vi "as2_startLogFile.vi"(4 "error in (no error)":errorcluster, 6 "Path In":path) -> (0 "error out":errorcluster, 2 "Path":path)   [LabVIEW 2013]
uses:
  <vilib>/Utility/file.llb/Write To Spreadsheet File (string).vi
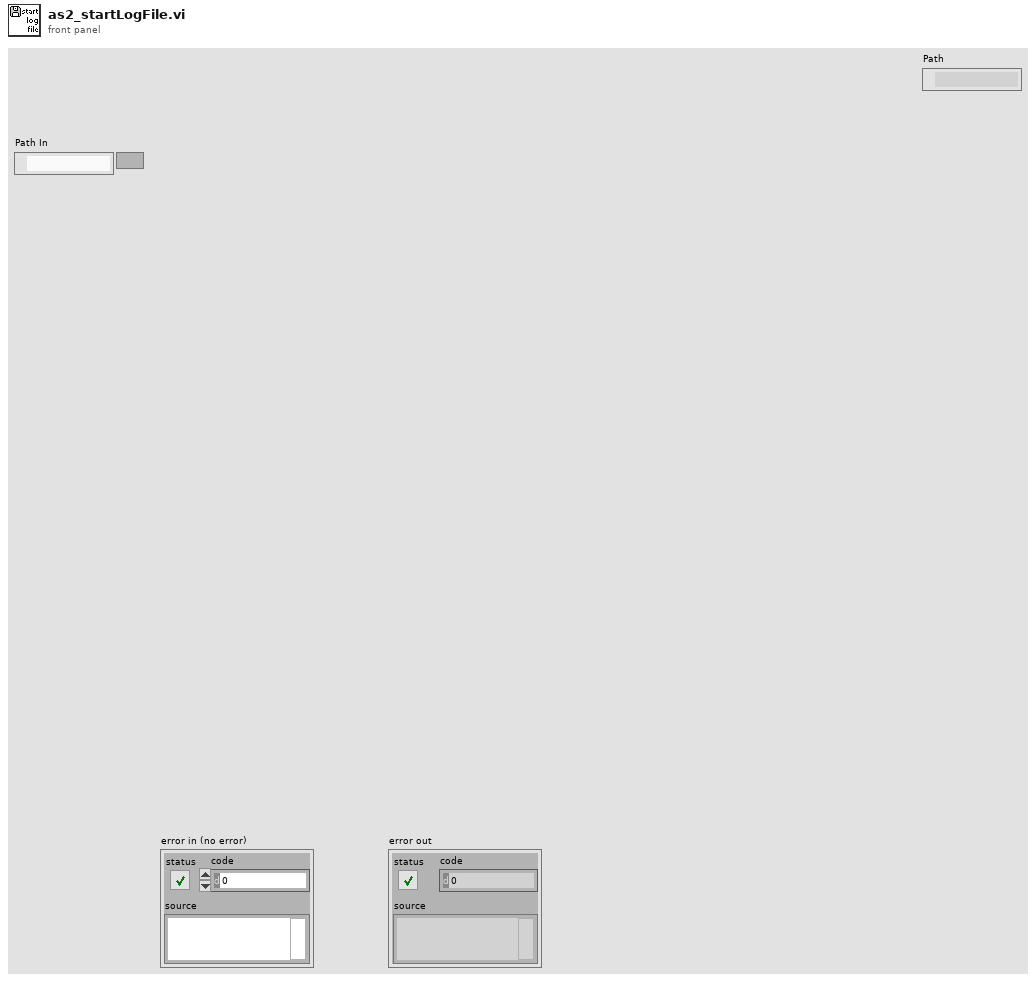
[diagram p1: front panel]
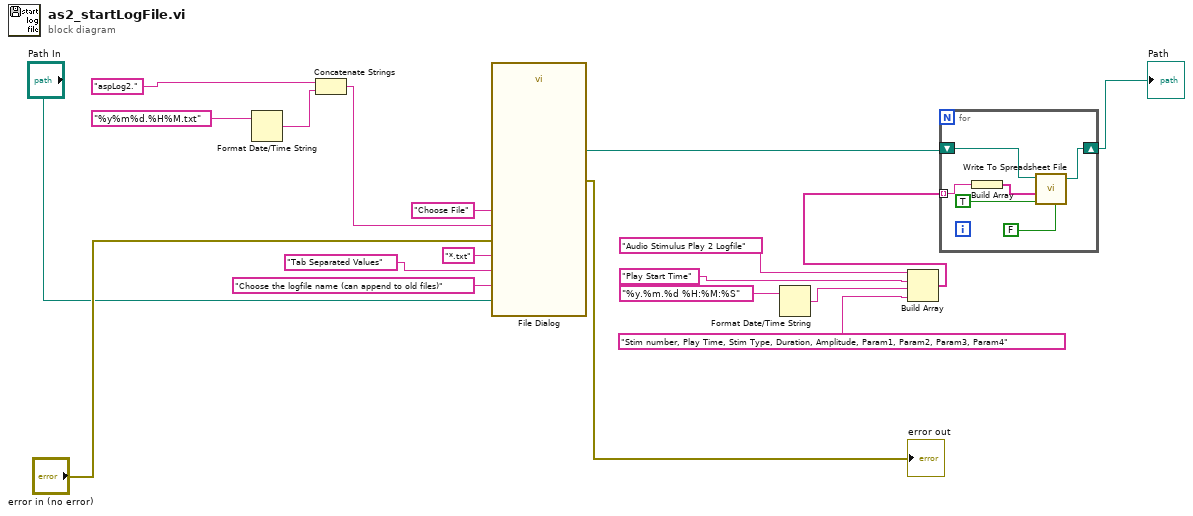
[diagram p0: block diagram]
diagram:
  n1 = Format Date/Time String(time format string (%c)="%y%m%d.%H%M.txt") -> (date/time string=w14:string)  [unwired: 2 in]
  n2 = Concatenate Strings("aspLog2.", w14) -> (w13:string)
  n3 = call "File Dialog"("start path"="Path In", "prompt"="Choose the logfile name (can append to old files)", "button label"="Choose File", "default name"=w13, "error in"="error in (no error)", "pattern (all files)"="*.txt", "pattern label"="Tab Separated Values") -> ("selected path"=w2:path, "error out"=→"error out":errorcluster)  [unwired: 5 in, 2 out]
  n4 = Format Date/Time String(time format string (%c)="%y.%m.%d %H:%M:%S") -> (date/time string=w4:string)  [unwired: 2 in]
  n5 = Build Array("Audio Stimulus Play 2 Logfile", "Play Start Time", w4, "Stim number, Play Time, Stim Type, Duration, Amplitude, Param1, Param2, Param3, Param4") -> (w5:string[])
  n6 = for {
    tunnel: w5 -> [w22] mode=indexing
    shift-right: [w24] -> w1
    shift-left: w2 -> [w23]
    n7 = Build Array(w22) -> (w21:string[])
    n8 = call-poly <vilib>:"Write To Spreadsheet File.vi"("transpose? (no:F)"=FALSE, "append to file? (new file:F)"=TRUE, "1D data"=w21, "file path (dialog if empty)"=w23) -> ("new file path (Not A Path if cancelled)"=w24:path)  [unwired: 4 in]
  }
  "Path" <- w1
